vi "ValidateToggleArray.vi"() -> (0 "Valid?":bool)   [LabVIEW 2012, in "FTC.lvlib" / "Remote Interface.lvlib"]
uses:
  Remote Interface.lvlib
  CLIB/CRef/CRef.lvlib
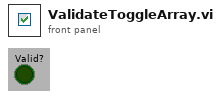
[diagram p1: front panel]
types:
  T1 = typedef "CRef.lvlib/I32 CReference.ctl" = cluster{"Generic CRef Address":u16, "Type":enum8{"Null", "Boolean", "U8", "I8", "U16", "I16", "U32", "I32", "U64", "I64", "Single", "Double", "Extended", "CSG", "CDB", "CXT", "Invalid Def", "U8(Def)", "I8(Def)", "U16(Def)", "I16(Def)", "U32(Def)", "I32(Def)"}}
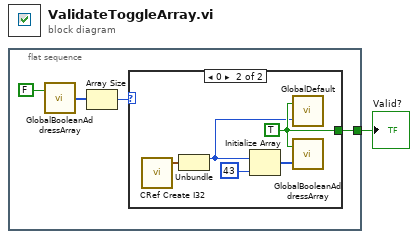
[diagram p0: block diagram]
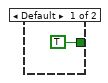
[diagram p2: hidden frame]
diagram:
  n1 = flat-sequence {
    tunnel: [w2] -> w1
    frame #0 {
      n2 = call "GlobalBooleanAddressArray.vi"("Write?"=FALSE) -> ("Array"=w4:u16[])  [unwired: 1 in]
      n3 = Array Size(array=w4) -> (size(s)=w3:i32)
      n4 = case shown="0" w3 {
        tunnel: [TRUE ("Write?") w9] -> w2
        frame Default {
        }
        frame 0 {
          w9 = TRUE ("Write?")
          n5 = call "CRef Create I32.vi"() -> ("I32 CReference"=w8:T1)  [unwired: 5 in]
          n6 = Unbundle(w8) -> ("Generic CRef Address"=w7:u16)  [unwired: 1 out]
          n7 = Initialize Array(w7, 43) -> (w10:u16[])
          n8 = call "GlobalDefault.vi"("Write Default"=w7, "Write?"=w9) -> ()  [unwired: 1 out]
          n9 = call "GlobalBooleanAddressArray.vi"("Write Array"=w10, "Write?"=w9) -> ()  [unwired: 1 out]
        }
      }
    }
  }
  "Valid?" <- w1
